vi "SeCrTs-DI Cumulative Sequence Check.vi"(6 "output cluster":T1, 9 "CDT":dbl, 10 "DI Data":bool, 11 "Numeric 2":i32) -> (1 "Failure case Seq":string, 2 "Boolean":bool, 3 "String":string)   [LabVIEW 2022 SP3]
panel:
  out "Numeric":i32
  out "number":dbl
  out "x >= y?":bool
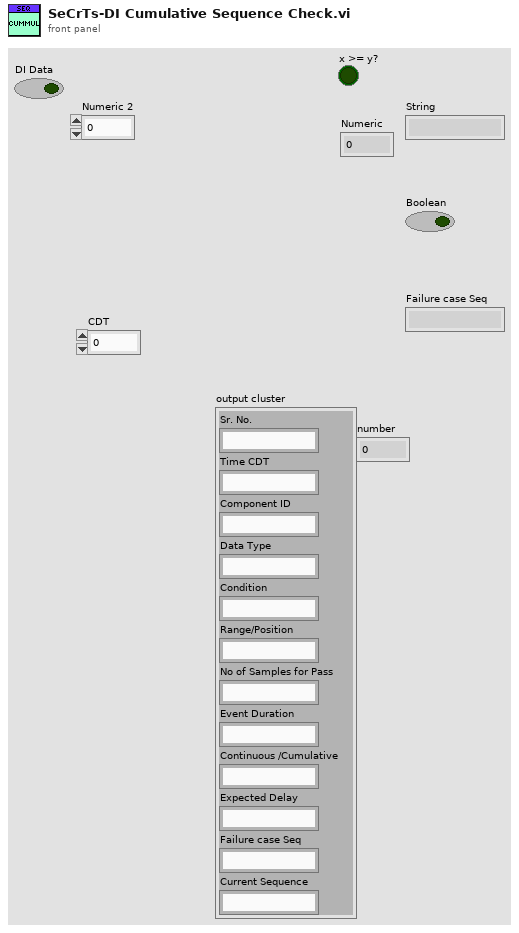
[diagram p1: front panel]
types:
  T1 = cluster{"Sr. No.":string, "Time CDT":string, "Component ID":string, "Data Type":string, "Condition":string, "Range/Position":string, "No of Samples for Pass":string, "Event Duration":string, "Continuous /Cumulative":string, "Expected Delay":string, "Failure case Seq":string, "Current Sequence":string}
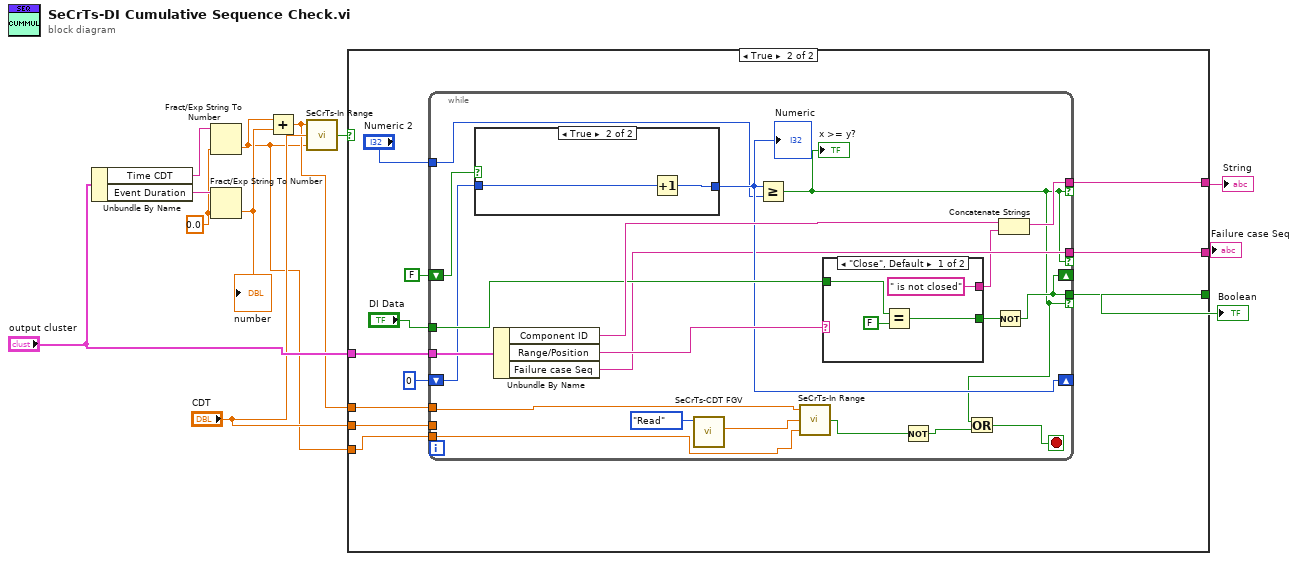
[diagram p0: block diagram]
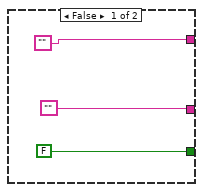
[diagram p2: hidden frame]
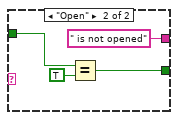
[diagram p3: hidden frame]
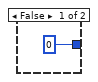
[diagram p4: hidden frame]
diagram:
  w6 = 0.0
  n1 = Unbundle By Name("output cluster") -> ("Time CDT"=w8:string, "Event Duration"=w7:string)
  n2 = Fract/Exp String To Number(string=w8, default (0 dbl)=w6) -> (number=w1:dbl)  [unwired: 2 in, 1 out]
  n3 = Fract/Exp String To Number(string=w7, default (0 dbl)=w6) -> (number=w9:dbl)  [unwired: 2 in, 1 out]
  "number" <- w9
  n4 = Add(x=w1, y=w9) -> (x+y=w2:dbl)
  n5 = call "SeCrTs-In Range.vi"("Min"=w1, "X"="CDT", "Max"=w2) -> ("In Range"=w3:bool)  [unwired: 2 in]
  n6 = case shown="True" w3 {
    tunnel: ["" ("Empty String Constant") w26] -> w12
    tunnel: ["" ("Empty String Constant") w25] -> w11
    tunnel: [FALSE w24] -> w10
    tunnel: "output cluster" -> [_ w21]
    tunnel: "CDT" -> [_ w20]
    tunnel: w2 -> [_ w17]
    tunnel: w1 -> [_ w16]
    frame False {
    }
    frame True {
      n7 = while {
        tunnel: w21 -> [w47]
        tunnel: [w44] -> w25 if=w28
        shift-right: [w38] -> _
        shift-left: FALSE -> [w41]
        tunnel: "DI Data" -> [w43]
        shift-right: [w40] -> _
        shift-left: 0 ("Numeric") -> [w42]
        tunnel: [w39] -> w26 if=w28
        tunnel: [w38] -> w24 if=w28
        tunnel: w20 -> [_]
        tunnel: "Numeric 2" -> [w35]
        tunnel: w17 -> [w32]
        tunnel: w16 -> [w31]
        stop <- w27 stop-if-true
        n8 = case shown="True" w41 {
          tunnel: [0 w58] -> w40
          tunnel: w42 -> [_ w57]
          frame False {
          }
          frame True {
            n9 = Increment(x=w57) -> (x+1=w58:i32)
          }
        }
        "Numeric" <- w40
        n10 = Unbundle By Name(w47) -> ("Component ID"=w45:string, "Range/Position"=w46:string, "Failure case Seq"=w39:string)
        n11 = call "SeCrTs-CDT FGV.vi"("Write/Read"=enum16{"Write", "Read"}."Read") -> ("CDT Out"=w33:dbl)  [unwired: 9 in, 1 out]
        n12 = Greater Or Equal?(x=w40, y=w35) -> (x >= y?=w28:bool)
        "x >= y?" <- w28
        n13 = call "SeCrTs-In Range.vi"("Min"=w31, "X"=w33, "Max"=w32) -> ("In Range"=w30:bool)  [unwired: 2 in]
        n14 = case shown="\"Close\", Default" w46 {
          tunnel: w43 -> [w50 w55]
          tunnel: [w48 w53] -> w37
          tunnel: [" is not closed" ("string") " is not opened" ("string")] -> w36
          frame "Close", Default {
            n15 = Equal?(x=w50, y=FALSE ("x")) -> (x = y?=w48:bool)
          }
          frame "Open" {
            n16 = Equal?(x=w55, y=TRUE ("x")) -> (x = y?=w53:bool)
          }
        }
        n17 = Not(x=w30) -> (.not. x?=w29:bool)
        n18 = Or(x=w28, y=w29) -> (x .or. y?=w27:bool)
        n19 = Not(x=w37) -> (.not. x?=w38:bool)
        n20 = Concatenate Strings(w45, w36) -> (w44:string)
      }
    }
  }
  "Failure case Seq" <- w12
  "String" <- w11
  "Boolean" <- w10
